vi "Cleanup.vi"(8 "error in (no error)":errorcluster, 11 "CRuleList in":refnum<class "CRuleList.lvclass">) -> (0 "error out":errorcluster, 3 "CRuleList out":refnum<class "CRuleList.lvclass">)   [LabVIEW 2020, in "DependencyInspection.lvlib" / "CRuleList.lvclass"]
uses:
  CRuleList.lvclass
  LabVIEWObjectInterfaces/IDependencyItemRule/IDependencyItemRule.lvclass
  RuleList.ctl
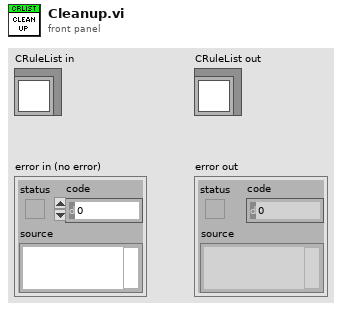
[diagram p1: front panel]
types:
  T1 = typedef "DependencyInspection.lvlib/CRuleList.lvclass/RuleList.ctl" = map{string, refnum<class "IDependencyItemRule.lvclass">}
  T2 = typedef "DependencyInspection.lvlib/CRuleList.lvclass/RuleListRef.ctl" = refnum<data-value>
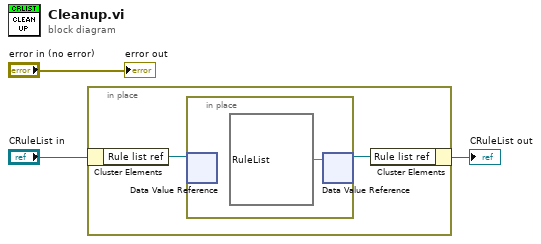
[diagram p0: block diagram]
diagram:
  n1 = in-place {
    n2 = in-place-cluster #1("CRuleList in") -> ("Rule list ref"=w5:T2)
    n3 = in-place {
      n4 = in-place-dvr #2(w5) -> ()  [unwired: 2 out]
      n5 = in-place-dvr #2(T1 {} ("data value")) -> (w4:T2)  [unwired: 1 out]
    }
    n6 = in-place-cluster #1("Rule list ref"=w4) -> (→"CRuleList out":refnum<class "CRuleList.lvclass">)
  }
  "error out" <- "error in (no error)"
